vi "GT_Update.vi"(2 "Axis in":T1=1 items=["Axis Control"=0, "Axis 1"=1, "Axis 2"=2, "Axis 3"=3, "Axis 4"=4, "Axis 5"=5, "Axis 6"=6, "Axis 7"=7, "Axis 8"=8, "Vector Space Control"=16, "Vector Space 1"=17, "Vector Space 2"=18, "Vector Space 3"=19, "Vector Space 4"=20], 3 "rtn_In":cluster{"rtn":i16, "Func":string}) -> (0 "Axis out":T1=1 items=["Axis Control"=0, "Axis 1"=1, "Axis 2"=2, "Axis 3"=3, "Axis 4"=4, "Axis 5"=5, "Axis 6"=6, "Axis 7"=7, "Axis 8"=8, "Vector Space Control"=16, "Vector Space 1"=17, "Vector Space 2"=18, "Vector Space 3"=19, "Vector Space 4"=20], 1 "rtn_Out":cluster{"rtn":i16, "Func":string})   [LabVIEW 2014]
uses:
  <vilib>/Motion/FlexMotion/CustomControls/CustomControls.llb/AxisOrVectorSpaceControl To Control.flx
  VC6/gts.dll
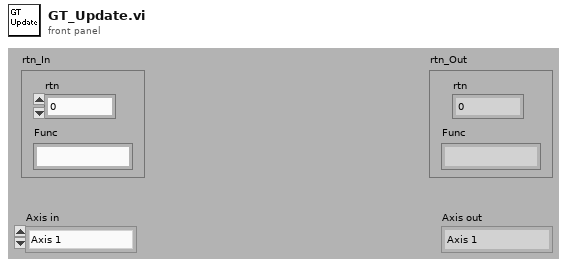
[diagram p1: front panel]
types:
  T1 = typedef "AxisOrVectorSpaceControl To Control.flx" = u16
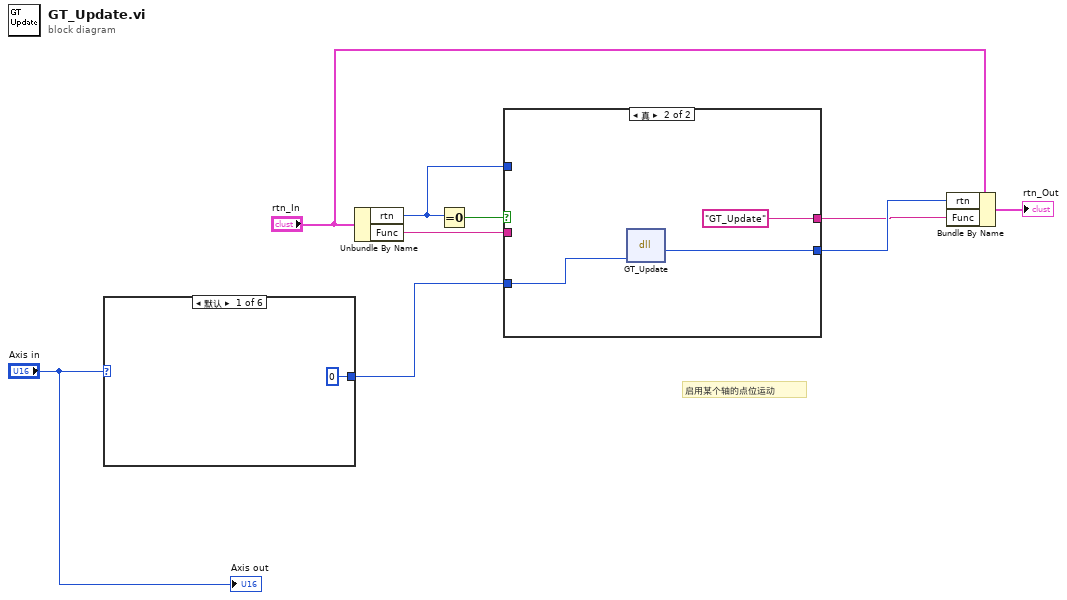
[diagram p0: block diagram]
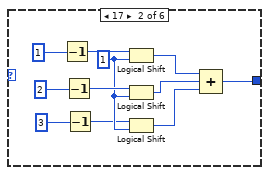
[diagram p2: hidden frame]
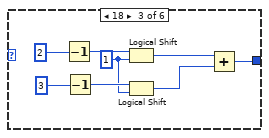
[diagram p3: hidden frame]
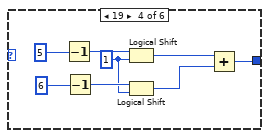
[diagram p4: hidden frame]
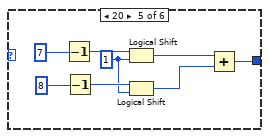
[diagram p5: hidden frame]
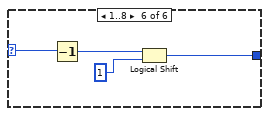
[diagram p6: hidden frame]
diagram:
  # "启用某个轴的点位运动"
  n1 = case shown="默认" "Axis in" {
    selector: "Axis in" -> [_ _ _ _ _ w49]
    tunnel: [0 w11 w23 w31 w39 w46] -> w2
    frame Default {
    }
    frame 17 {
      w17 = 1 ("x")
      n2 = Decrement(x=1) -> (x-1=w21:i32)
      n3 = Decrement(x=2) -> (x-1=w18:i32)
      n4 = Decrement(x=3) -> (x-1=w15:i32)
      n5 = Logical Shift(y=w21, x=w17) -> (x << y=w14:i32)
      n6 = Logical Shift(y=w18, x=w17) -> (x << y=w13:i32)
      n7 = Logical Shift(y=w15, x=w17) -> (x << y=w12:i32)
      n8 = Compound Arithmetic op=unknown(w14, w13, w12) -> (w11:i32)
    }
    frame 18 {
      w22 = 1 ("x")
      n9 = Decrement(x=2) -> (x-1=w28:i32)
      n10 = Decrement(x=3) -> (x-1=w26:i32)
      n11 = Logical Shift(y=w28, x=w22) -> (x << y=w25:i32)
      n12 = Logical Shift(y=w26, x=w22) -> (x << y=w24:i32)
      n13 = Add(x=w25, y=w24) -> (x+y=w23:i32)
    }
    frame 19 {
      w30 = 1 ("x")
      n14 = Decrement(x=5) -> (x-1=w36:i32)
      n15 = Decrement(x=6) -> (x-1=w34:i32)
      n16 = Logical Shift(y=w36, x=w30) -> (x << y=w33:i32)
      n17 = Logical Shift(y=w34, x=w30) -> (x << y=w32:i32)
      n18 = Add(x=w33, y=w32) -> (x+y=w31:i32)
    }
    frame 20 {
      w38 = 1 ("x")
      n19 = Decrement(x=7) -> (x-1=w44:i32)
      n20 = Decrement(x=8) -> (x-1=w42:i32)
      n21 = Logical Shift(y=w44, x=w38) -> (x << y=w41:i32)
      n22 = Logical Shift(y=w42, x=w38) -> (x << y=w40:i32)
      n23 = Add(x=w41, y=w40) -> (x+y=w39:i32)
    }
    frame 1..8 {
      n24 = Decrement(x=w49) -> (x-1=w48:T1)
      n25 = Logical Shift(y=w48, x=1) -> (x << y=w46:i32)
    }
  }
  n26 = Unbundle By Name("rtn_In") -> ("rtn"=w3:i16, "Func"=w8:string)
  n27 = Equal To 0?(x=w3) -> (x = 0?=w9:bool)
  n28 = case shown="真" w9 {
    tunnel: w8 -> [w51 _]
    tunnel: [w50 w54] -> w5
    tunnel: [w51 "GT_Update" ("Func")] -> w4
    tunnel: w3 -> [w50 _]
    tunnel: w2 -> [_ w52]
    frame False {
    }
    frame True {
      n29 = dll-call lib="PTH2Fabs DNewGTS AC-800LWin7版源程序-20170926gts85VC6gts.dll" fn="GT_Update"("Mask"=w52) -> ("rtn"=w54:i16)  [unwired: 4 in, 2 out]
    }
  }
  n30 = Bundle By Name(cluster="rtn_In", "rtn"=w5, "Func"=w4) -> (→"rtn_Out":cluster{"rtn":i16, "Func":string})
  "Axis out" <- "Axis in"
